vi "Read Escaped.vi"(8 "Error In":errorcluster, 11 "Variable In":refnum<class "Variable.lvclass">) -> (0 "Error Out":errorcluster, 2 "Escaped":bool, 3 "Variable Out":refnum<class "Variable.lvclass">)   [LabVIEW 2018, in "Toolkit.lvlib" / "Nodes.lvlib" / "Variable.lvclass"]
uses:
  Variable.lvclass
  Variable.lvclass/Variable.ctl
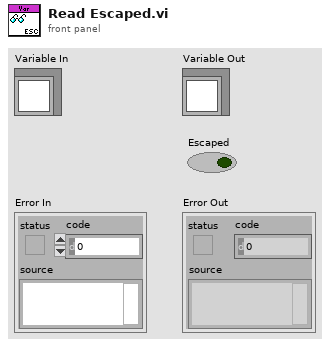
[diagram p1: front panel]
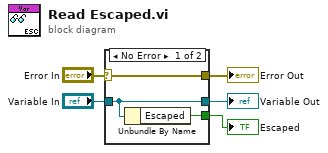
[diagram p0: block diagram]
diagram:
  n1 = case shown="No Error" "Error In" {
    selector: "Error In" -> [w8 w9]
    tunnel: [w8 w9] -> w4
    tunnel: [w7 w10] -> w2
    tunnel: "Variable In" -> [w7 w10]
    tunnel: [w6 _] -> w1
    frame No Error {
      n2 = Unbundle By Name(w7) -> ("Escaped"=w6:bool)
    }
    frame Error {
    }
  }
  "Error Out" <- w4
  "Variable Out" <- w2
  "Escaped" <- w1
